vi "GoToHeight-C.vi"(11 "Params":string[][](array[string])) -> ()   [LabVIEW 2018]
uses:
  Framework/Robot Global Data.vi
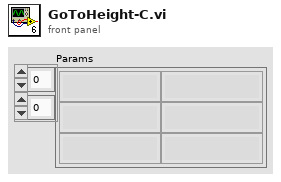
[diagram p1: front panel]
types:
  T1 = typedef "Command Status Info.ctl" = cluster{"Name":string, "Status":T2, "notifier out":T3}
  T2 = typedef "Completion Status.ctl" = enum16{"Successful", "Aborted", "Incomplete"}
  T3 = typedef "Completion Notifier.ctl" = refnum<notifier>
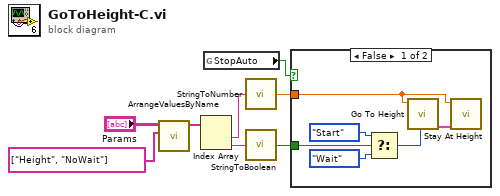
[diagram p0: block diagram]
diagram:
  n1 = call "ArrangeValuesByName.vi"("Names"=string[] ["Height", "NoWait"], "Names/Values in"="Params") -> ("Values Out"=w3:string[])  [unwired: 9 in]
  n2 = Index Array(array=w3) -> (element #1=w2:string, element #2=w1:string)  [unwired: 2 in]
  n3 = global read "Robot Global Data.vi" "StopAuto"() -> (w8:bool)
  n4 = call "StringToNumber.vi"("String"=w2) -> ("Output"=w7:dbl)
  n5 = call "StringToBoolean.vi"("String"=w1) -> ("Output"=w6:bool)
  n6 = case shown="False" w8 {
    tunnel: w7 -> [w9 _]
    tunnel: w6 -> [w12 _]
    frame False {
      n7 = Select(t=enum16{"Start", "Wait"}."Start" ("Synchronization"), s=w12, f=enum16{"Start", "Wait"}."Wait" ("Synchronization")) -> (s? t:f=w11:enum16{"Start", "Wait"})
      n8 = call "Go To Height.vi"("Synchronization"=w11, "Height"=w9) -> ("Command Info Out"=w10:T1)  [unwired: 9 in]
      n9 = call "Stay At Height.vi"("Command Info In"=w10, "Height"=w9) -> ()  [unwired: 9 in, 1 out]
    }
    frame True {
    }
  }
